vi "startReadSetDuration.vi"(8 "error in (no error)":errorcluster, 10 "ElectrometerController in":refnum<class "ElectrometerController.lvclass">, 11 "ReadyState in":refnum<class "ReadyState.lvclass">) -> (0 "error out":errorcluster, 2 "ElectrometerController out":refnum<class "ElectrometerController.lvclass">, 3 "ReadyState out":refnum<class "ReadyState.lvclass">)   [LabVIEW 2016, in "ReadyState.lvclass"]
uses:
  ReadyState.lvclass
  ElectrometerController/ElectrometerController.lvclass
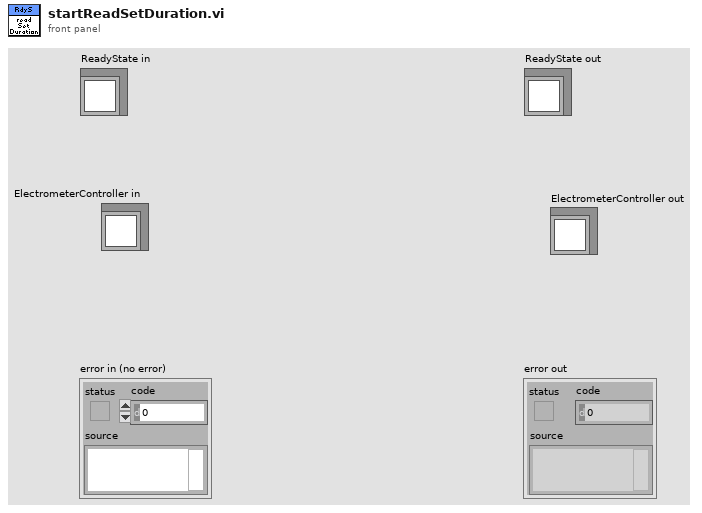
[diagram p1: front panel]
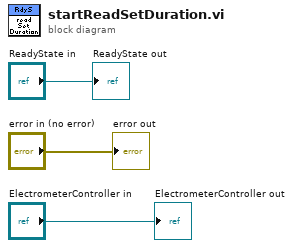
[diagram p0: block diagram]
diagram:
  "error out" <- "error in (no error)"
  "ReadyState out" <- "ReadyState in"
  "ElectrometerController out" <- "ElectrometerController in"
